vi "OutputSwerveDrive2.vi"() -> ()   [LabVIEW 2019]
doc: "This VI runs feedback and feedforward control loops, manages safety interlocks, and sends commands to the swerve drive motors."
uses:
  <vilib>/Rock Robotics/WPI/ThirdParty/Phoenix-LabVIEW/Motor Controller/Controls/CTRE_Phoenix_MotorControl_SupplyCurrentLimitConfiguration.ctl
  <vilib>/Rock Robotics/WPI/ThirdParty/Phoenix-LabVIEW/Motor Controller/Controls/CTRE_Phoenix_MotorControl_ControlMode.ctl
  <vilib>/Rock Robotics/WPI/Solenoid/WPI_SolenoidValue.ctl
  4c0f1fb3-de9e-41af-b613-55c778746a69.vi
  9255c0bb-7061-46f3-9b12-3c6a122af16e.vi
  1feddb54-1091-429e-8d95-9769f01e3028.vi
  eec0778c-44f4-445b-8f09-fbe21d33a92f.vi
  5bc46b9e-4d4b-4873-ab3e-533fd441fb60.vi
  9914bed3-0d1c-4b06-b050-22aab9a27a8c.vi
  outputs.vi
  sensors.vi
  refnums.vi
  GRNF_CTREMotor.vi
  robotprofile.vi
  <vilib>/Rock Robotics/WPI/ThirdParty/Phoenix-LabVIEW/Motor Controller/Get/CTRE_Phoenix_MotorController_GetVoltage.vi
  <vilib>/Rock Robotics/WPI/ThirdParty/Phoenix-LabVIEW/Motor Controller/Get/CTRE_Phoenix_MotorController_GetSelectedSensorData.vi
  GRNF_GenericSolenoid.vi
  dsdata.vi
  TAI_Solenoid.vi
  <vilib>/Rock Robotics/WPI/Solenoid/WPI_SolenoidSetEnum.vi
  TAI_Motor.vi
panel:
  in  "Time Below Speed (ms)":u32=500
  in  "Time Above Speed (ms)":u32=500
  in  "Switch to Low Gear (rpm)":dbl=2000.0
  in  "Switch to High Gear (rpm)":dbl=3000.0
  in  "Plotting":T1(ring)
  in  "Falcon PID":T2={"P Gain"=0.1, "I Gain"=0.0, "D Gain"=0.0, "F Gain"=0.045, "I Zone"=200.0, "Min Output"=-1.0, "Max Output"=1.0} {"Max Output" min=-1.0 max=1.0 step=0.01; "Min Output" min=-1.0 max=1.0 step=0.01; "I Zone" step=0.01; "F Gain" step=0.01; "D Gain" step=0.01; "I Gain" step=0.01; "P Gain" min=0.0 step=0.01}
  out "Controller Summary":T3(graph)
  in  "Max Speed (rpm)":dbl=6400.0
  in  "Min Speed (rpm)":dbl=10.0
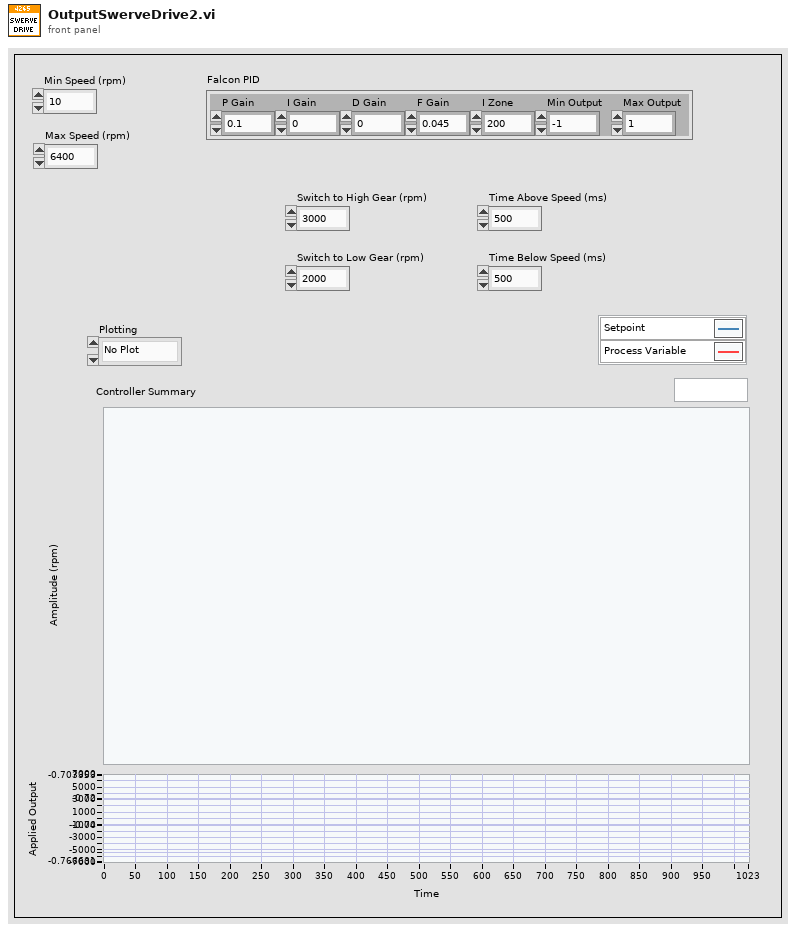
[diagram p1: front panel]
types:
  T1 = enum16{"No Plot", "Module 0", "Module 1", "Module 2", "Module 3"}
  T2 = cluster{"P Gain":dbl, "I Gain":dbl, "D Gain":dbl, "F Gain":dbl, "I Zone":dbl, "Min Output":dbl, "Max Output":dbl}
  T3 = cluster{"Sensor Velocity":dbl, "Setpoint":dbl, "Applied Output":dbl}
  T4 = typedef "CTRE_Phoenix_MotorControl_ControlMode.ctl" = u16
  T5 = typedef "CTRE_Phoenix_MotorControl_SupplyCurrentLimitConfiguration.ctl" = cluster{"Enable?":bool, "Current Limit":dbl, "Threshold Current":dbl, "Threshold Time":dbl}
  T6 = typedef "WPI_MotorControlDeviceRef.ctl" = cluster{"DeviceStatus":errorcluster, "Type":T7, "PWM":cluster{"PWM Channel":T8, "DeadBand":T9}, "CAN":cluster{"Device Number":u8, "SetOutput VI Ref":variant, "GetOutput VI Ref":variant, "Enable VI Ref":variant, "Disable VI Ref":variant, "Data":variant}, "Invert":bool, "DIO PWM":cluster{"PWM \"Enable\" Channel":T8, "DIOChannel":T10, "PWM Rate":dbl}}
  T7 = typedef "WPI_MotorControlType.ctl" = enum16{"PWM", "CAN", "DIO PWM"}
  T8 = typedef "FPGA_DIOPWMChannel.ctl" = enum8{"PWM 0", "PWM 1", "PWM 2", "PWM 3", "PWM 4", "PWM 5", "PWM 6", "PWM 7", "PWM 8", "PWM 9", "PWM MXP 0", "PWM MXP 1", "PWM MXP 2", "PWM MXP 3", "PWM MXP 4", "PWM MXP 5", "PWM MXP 6", "PWM MXP 7", "PWM MXP 8", "PWM MXP 9", "Invalid"}
  T9 = typedef "WPI_PWMDeadband.ctl" = cluster{"Name":string, "maxPositivePwm":i32, "minPositivePwm":i32, "centerPwm":i32, "maxNegativePwm":i32, "minNegativePwm":i32, "angularRange":u16}
  T10 = typedef "FPGA_DIOChannel.ctl" = enum8{"DIO 0", "DIO 1", "DIO 2", "DIO 3", "DIO 4", "DIO 5", "DIO 6", "DIO 7", "DIO 8", "DIO 9", "DIO MXP 0", "DIO MXP 1", "DIO MXP 2", "DIO MXP 3", "DIO MXP 4", "DIO MXP 5", "DIO MXP 6", "DIO MXP 7", "DIO MXP 8", "DIO MXP 9", "DIO MXP 10", "DIO MXP 11", "DIO MXP 12", "DIO MXP 13", "DIO MXP 14", "DIO MXP 15", "SPI Port CS1", "SPI Port CS2", "SPI Port CS3", "SPI Port MISO", "SPI Port MOSI", "Invalid"}
  T11 = cluster{"P Gain":bool, "I Gain":bool, "D Gain":bool, "F Gain":bool, "I Zone":bool, "Min Output":bool, "Max Output":bool}
  T12 = typedef "WPI_SolenoidValue.ctl" = enum16{"Off", "On", "Forward", "Reverse"}
  T13 = typedef "WPI_SolenoidDevRef.ctl" = cluster{"DevStatus":errorcluster, "Pneumatics Control Module":u8, "Forward Solenoid Channel":T14, "Reverse Solenoid Channel":T14}
  T14 = typedef "WPI_SolenoidChannel.ctl" = enum8{"Solenoid 0", "Solenoid 1", "Solenoid 2", "Solenoid 3", "Solenoid 4", "Solenoid 5", "Solenoid 6", "Solenoid 7", "Invalid"}
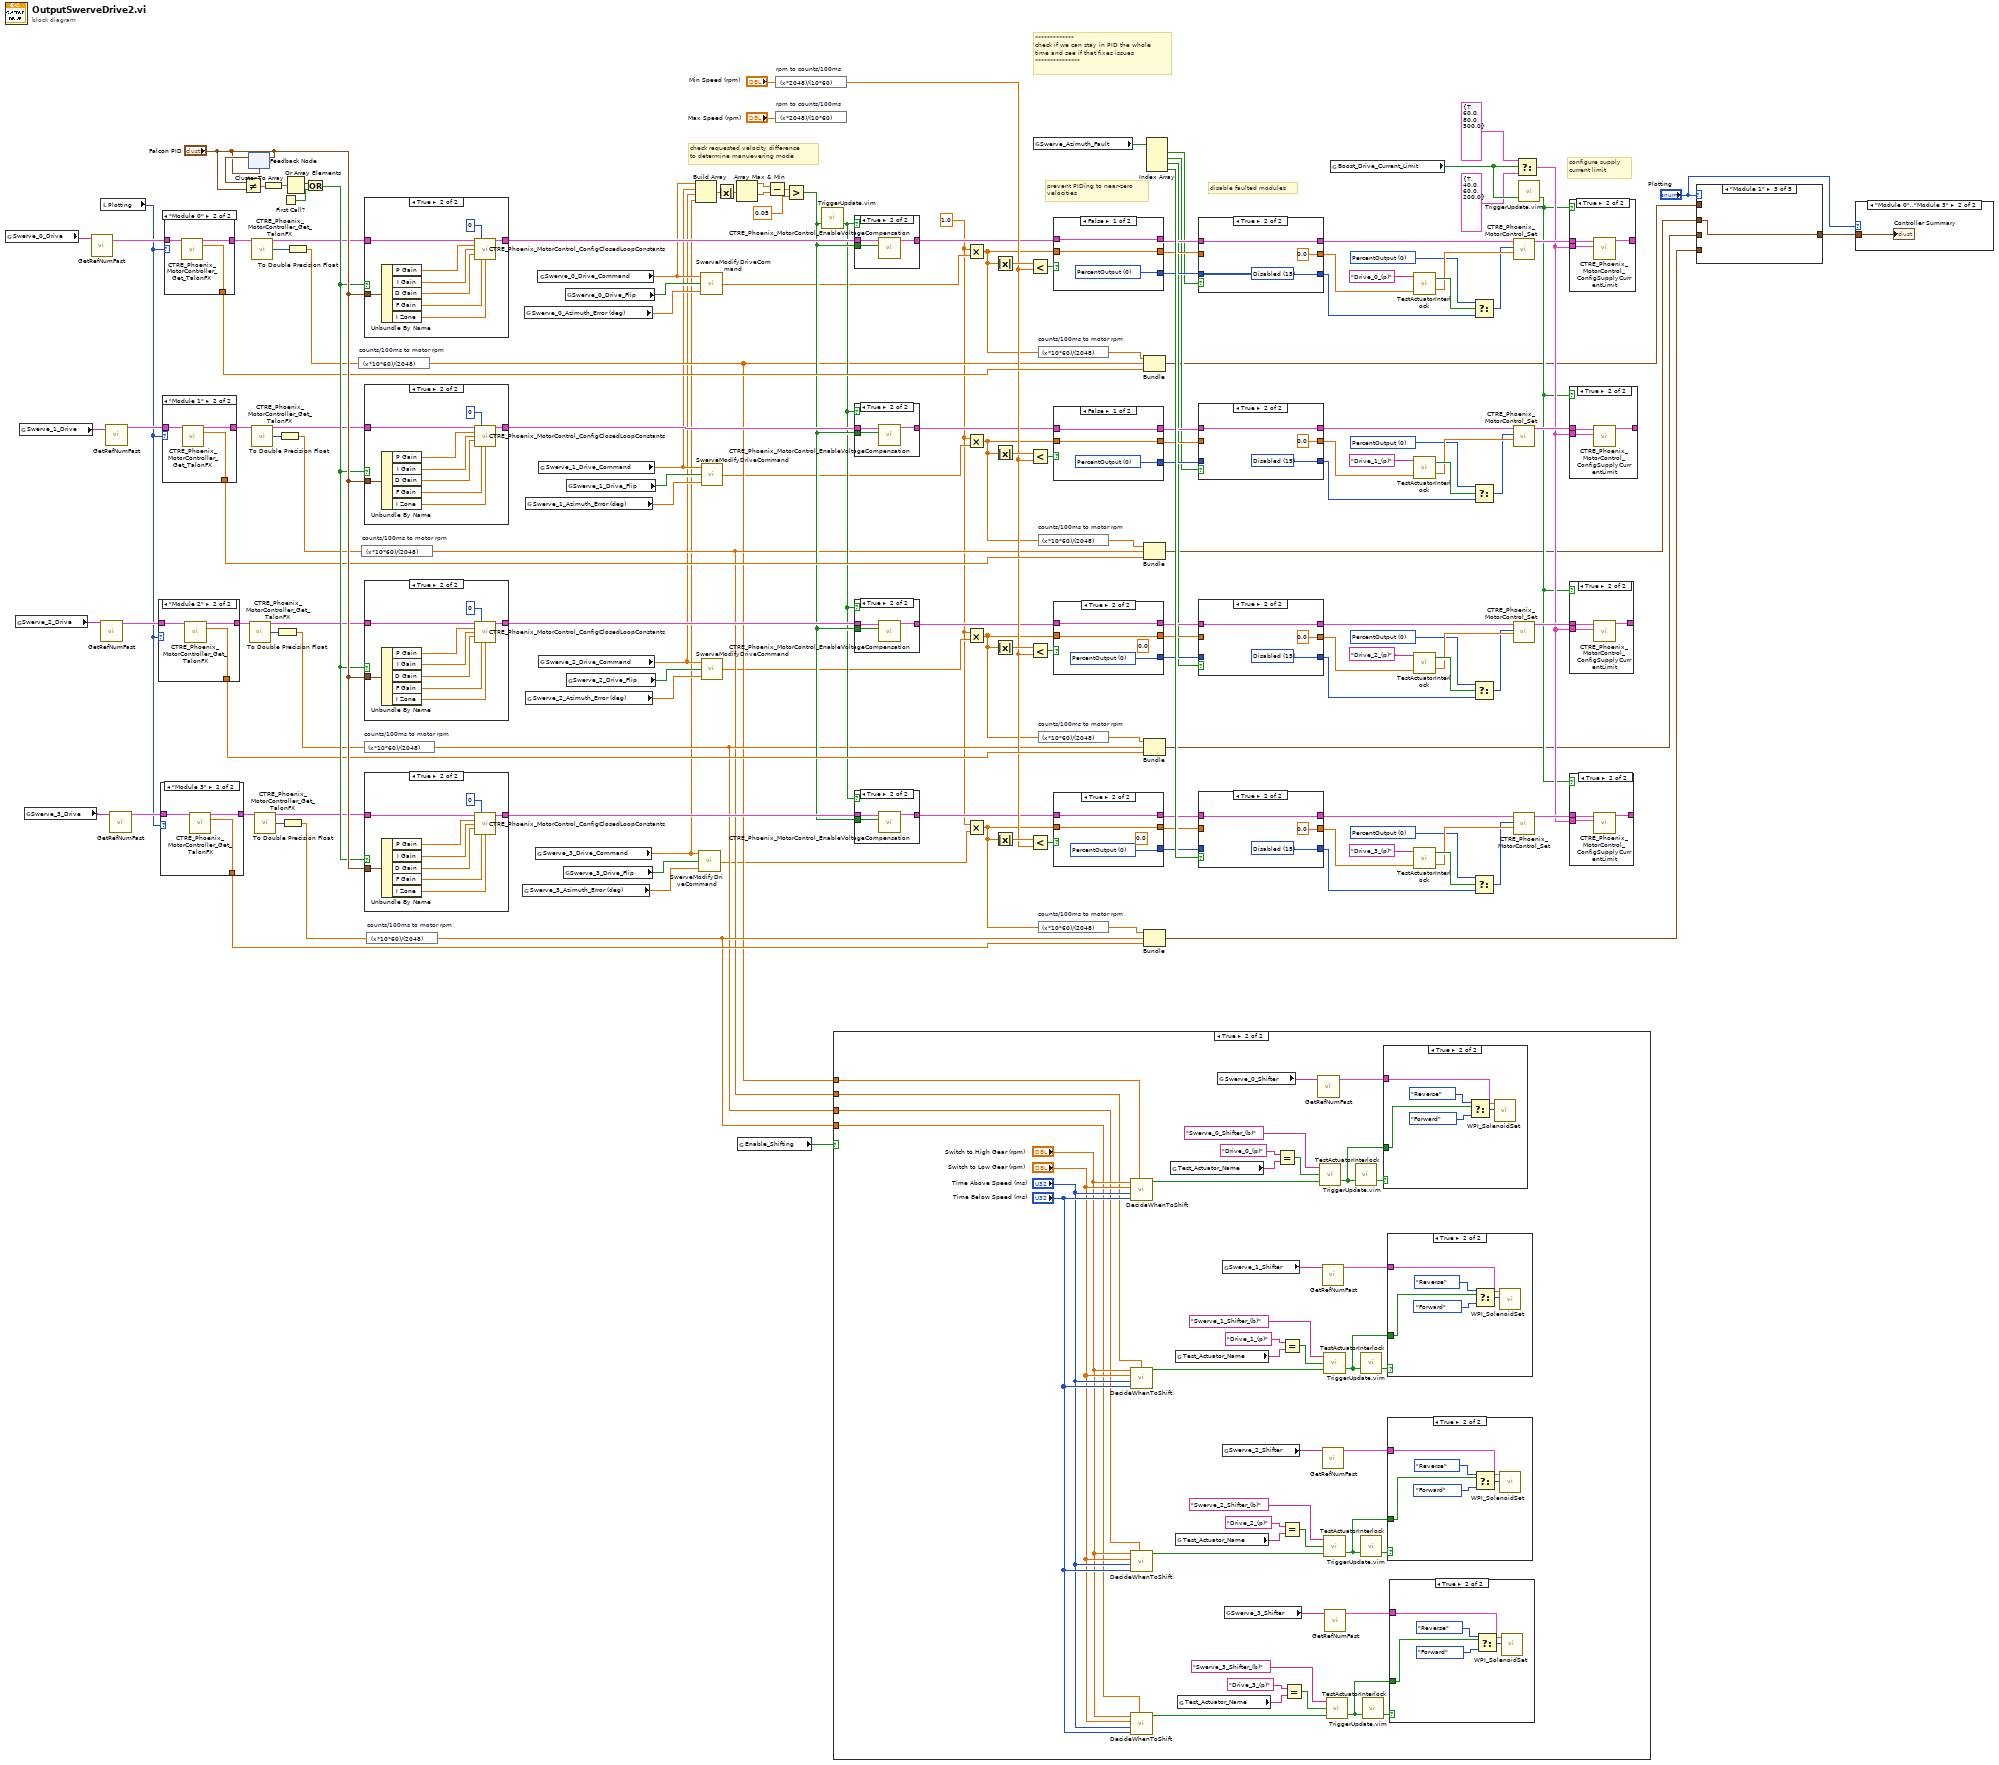
[diagram p0: block diagram]
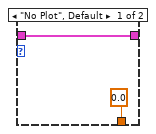
[diagram p2: hidden frame]
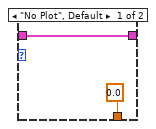
[diagram p3: hidden frame]
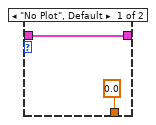
[diagram p4: hidden frame]
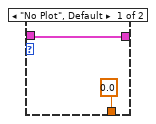
[diagram p5: hidden frame]
diagram:
  w1 = 1.0 ("x")
  w94 = T4 0 items=["PercentOutput"=0, "Position"=1, "Velocity"=2, "Current"=3, "Follower"=5, "MotionProfile"=6, "MotionMagic"=7, "MotionProfileArc"=10, "Disabled"=15] ("Control Mode")
  w108 = T4 0 items=["PercentOutput"=0, "Position"=1, "Velocity"=2, "Current"=3, "Follower"=5, "MotionProfile"=6, "MotionMagic"=7, "MotionProfileArc"=10, "Disabled"=15] ("Control Mode")
  w122 = T4 0 items=["PercentOutput"=0, "Position"=1, "Velocity"=2, "Current"=3, "Follower"=5, "MotionProfile"=6, "MotionMagic"=7, "MotionProfileArc"=10, "Disabled"=15] ("Control Mode")
  w136 = T4 0 items=["PercentOutput"=0, "Position"=1, "Velocity"=2, "Current"=3, "Follower"=5, "MotionProfile"=6, "MotionMagic"=7, "MotionProfileArc"=10, "Disabled"=15] ("Control Mode")
  # "*************\ncheck if we can stay in PID the whole \ntime and see if that fixes issues\n***************"
  # "check requested velocity difference\nto determine manuevering mode"
  # "configure supply\ncurrent limit"
  # "disable faulted modules"
  # "prevent PIDing to near-zero\nvelocities"
  n1 = global read "refnums.vi" "Swerve_0_Drive"() -> (w105:string)
  n2 = global read "refnums.vi" "Swerve_2_Drive"() -> (w133:string)
  n3 = global read "refnums.vi" "Swerve_1_Drive"() -> (w119:string)
  n4 = global read "refnums.vi" "Swerve_3_Drive"() -> (w143:string)
  n5 = call-poly "GetRefNumFast.vi"("RefNum Name"=w105) -> ("Device Reference"=w68:T6)  [unwired: 5 in, 1 out]
  n6 = local read "Plotting"() -> (w18:T1)
  n7 = call-poly "GetRefNumFast.vi"("RefNum Name"=w133) -> ("Device Reference"=w74:T6)  [unwired: 5 in, 1 out]
  n8 = call-poly "GetRefNumFast.vi"("RefNum Name"=w119) -> ("Device Reference"=w71:T6)  [unwired: 5 in, 1 out]
  n9 = call-poly "GetRefNumFast.vi"("RefNum Name"=w143) -> ("Device Reference"=w76:T6)  [unwired: 5 in, 1 out]
  n10 = case shown="\"Module 2\"" w18 {
    tunnel: [0.0 ("Percent Output") w162] -> w75
    tunnel: w74 -> [w159 w161]
    tunnel: [w159 w160] -> w21
    frame "No Plot", Default {
    }
    frame "Module 2" {
      n11 = call-poly <vilib>:"CTRE_Phoenix_MotorController_Get_TalonFX.vi"("PhoenixMotorControlDevRef"=w161) -> ("PhoenixMotorControlDevRef"=w160:T6, "Percent Output"=w162:dbl)  [unwired: 10 in, 3 out]
    }
  }
  n12 = case shown="\"Module 3\"" w18 {
    tunnel: [0.0 ("Percent Output") w167] -> w78
    tunnel: w76 -> [w164 w166]
    tunnel: [w164 w165] -> w19
    frame "No Plot", Default {
    }
    frame "Module 3" {
      n13 = call-poly <vilib>:"CTRE_Phoenix_MotorController_Get_TalonFX.vi"("PhoenixMotorControlDevRef"=w166) -> ("PhoenixMotorControlDevRef"=w165:T6, "Percent Output"=w167:dbl)  [unwired: 10 in, 3 out]
    }
  }
  n14 = case shown="\"Module 1\"" w18 {
    tunnel: [0.0 ("Percent Output") w172] -> w72
    tunnel: w71 -> [w169 w171]
    tunnel: [w169 w170] -> w23
    frame "No Plot", Default {
    }
    frame "Module 1" {
      n15 = call-poly <vilib>:"CTRE_Phoenix_MotorController_Get_TalonFX.vi"("PhoenixMotorControlDevRef"=w171) -> ("PhoenixMotorControlDevRef"=w170:T6, "Percent Output"=w172:dbl)  [unwired: 10 in, 3 out]
    }
  }
  n16 = case shown="\"Module 0\"" w18 {
    tunnel: [0.0 ("Percent Output") w177] -> w69
    tunnel: w68 -> [w174 w176]
    tunnel: [w174 w175] -> w25
    frame "No Plot", Default {
    }
    frame "Module 0" {
      n17 = call-poly <vilib>:"CTRE_Phoenix_MotorController_Get_TalonFX.vi"("PhoenixMotorControlDevRef"=w176) -> ("PhoenixMotorControlDevRef"=w175:T6, "Percent Output"=w177:dbl)  [unwired: 10 in, 3 out]
    }
  }
  n18 = feedback #1("Falcon PID") -> (w142:T2)
  n19 = Not Equal?(x=w142, y="Falcon PID") -> (x != y?=w147:T11)
  n20 = feedback-in #1("Falcon PID") -> ()
  n21 = call-poly <vilib>:"CTRE_Phoenix_MotorController_Get_TalonFX.vi"("PhoenixMotorControlDevRef"=w21) -> ("PhoenixMotorControlDevRef"=w32:T6, "Velocity (Raw Sensor Units per 100 ms)"=w22:i32)  [unwired: 11 in, 2 out]
  n22 = call-poly <vilib>:"CTRE_Phoenix_MotorController_Get_TalonFX.vi"("PhoenixMotorControlDevRef"=w25) -> ("PhoenixMotorControlDevRef"=w37:T6, "Velocity (Raw Sensor Units per 100 ms)"=w26:i32)  [unwired: 11 in, 2 out]
  n23 = call-poly <vilib>:"CTRE_Phoenix_MotorController_Get_TalonFX.vi"("PhoenixMotorControlDevRef"=w23) -> ("PhoenixMotorControlDevRef"=w34:T6, "Velocity (Raw Sensor Units per 100 ms)"=w24:i32)  [unwired: 11 in, 2 out]
  n24 = call-poly <vilib>:"CTRE_Phoenix_MotorController_Get_TalonFX.vi"("PhoenixMotorControlDevRef"=w19) -> ("PhoenixMotorControlDevRef"=w30:T6, "Velocity (Raw Sensor Units per 100 ms)"=w20:i32)  [unwired: 11 in, 2 out]
  n25 = Cluster To Array(cluster=w147) -> (array=w148:bool[])
  n26 = To Double Precision Float(number=w22) -> (double precision float=w33:dbl)
  n27 = To Double Precision Float(number=w24) -> (double precision float=w35:dbl)
  n28 = First Call?() -> (First Call?: T/F=w145:bool)
  n29 = To Double Precision Float(number=w20) -> (double precision float=w31:dbl)
  n30 = Or Array Elements(Boolean array=w148) -> (logical OR=w146:bool)
  n31 = To Double Precision Float(number=w26) -> (double precision float=w36:dbl)
  n32 = Or(x=w146, y=w145) -> (x .or. y?=w90:bool)
  n33 = expression code="(x*10*60)/(2048)" "counts/100ms to motor rpm"(w36) -> (w27:dbl)
  n34 = expression code="(x*10*60)/(2048)" "counts/100ms to motor rpm"(w35) -> (w28:dbl)
  n35 = expression code="(x*10*60)/(2048)" "counts/100ms to motor rpm"(w33) -> (w29:dbl)
  n36 = case shown="True" w90 {
    tunnel: "Falcon PID" -> [_ w186]
    tunnel: [w178 w187] -> w48
    tunnel: w37 -> [w178 w179]
    frame False {
    }
    frame True {
      n37 = Unbundle By Name(w186) -> ("P Gain"=w185:dbl, "I Gain"=w184:dbl, "D Gain"=w183:dbl, "F Gain"=w182:dbl, "I Zone"=w181:dbl)
      n38 = call <vilib>:"CTRE_Phoenix_MotorControl_ConfigClosedLoopConstants.vi"("PhoenixMotorControlDevRef"=w179, "slotIdx"=0, "P"=w185, "I"=w184, "D"=w183, "F"=w182, "I Zone"=w181) -> ("PhoenixMotorControlDevRef"=w187:T6)  [unwired: 7 in, 1 out]
    }
  }
  n39 = case shown="True" w90 {
    tunnel: w34 -> [w188 w196]
    tunnel: "Falcon PID" -> [_ w195]
    tunnel: [w188 w197] -> w46
    frame False {
    }
    frame True {
      n40 = Unbundle By Name(w195) -> ("P Gain"=w189:dbl, "I Gain"=w194:dbl, "D Gain"=w193:dbl, "F Gain"=w192:dbl, "I Zone"=w191:dbl)
      n41 = call <vilib>:"CTRE_Phoenix_MotorControl_ConfigClosedLoopConstants.vi"("PhoenixMotorControlDevRef"=w196, "slotIdx"=0, "P"=w189, "I"=w194, "D"=w193, "F"=w192, "I Zone"=w191) -> ("PhoenixMotorControlDevRef"=w197:T6)  [unwired: 7 in, 1 out]
    }
  }
  n42 = case shown="True" w90 {
    tunnel: w32 -> [w198 w206]
    tunnel: "Falcon PID" -> [_ w205]
    tunnel: [w198 w207] -> w44
    frame False {
    }
    frame True {
      n43 = Unbundle By Name(w205) -> ("P Gain"=w204:dbl, "I Gain"=w203:dbl, "D Gain"=w202:dbl, "F Gain"=w201:dbl, "I Zone"=w200:dbl)
      n44 = call <vilib>:"CTRE_Phoenix_MotorControl_ConfigClosedLoopConstants.vi"("PhoenixMotorControlDevRef"=w206, "slotIdx"=0, "P"=w204, "I"=w203, "D"=w202, "F"=w201, "I Zone"=w200) -> ("PhoenixMotorControlDevRef"=w207:T6)  [unwired: 7 in, 1 out]
    }
  }
  n45 = case shown="True" w90 {
    tunnel: w30 -> [w208 w216]
    tunnel: "Falcon PID" -> [_ w215]
    tunnel: [w208 w217] -> w42
    frame False {
    }
    frame True {
      n46 = Unbundle By Name(w215) -> ("P Gain"=w214:dbl, "I Gain"=w213:dbl, "D Gain"=w212:dbl, "F Gain"=w211:dbl, "I Zone"=w210:dbl)
      n47 = call <vilib>:"CTRE_Phoenix_MotorControl_ConfigClosedLoopConstants.vi"("PhoenixMotorControlDevRef"=w216, "slotIdx"=0, "P"=w214, "I"=w213, "D"=w212, "F"=w211, "I Zone"=w210) -> ("PhoenixMotorControlDevRef"=w217:T6)  [unwired: 7 in, 1 out]
    }
  }
  n48 = expression code="(x*10*60)/(2048)" "counts/100ms to motor rpm"(w31) -> (w63:dbl)
  n49 = global read "outputs.vi" "Swerve_3_Azimuth_Error (deg)"() -> (w4:dbl)
  n50 = global read "outputs.vi" "Swerve_0_Azimuth_Error (deg)"() -> (w15:dbl)
  n51 = global read "outputs.vi" "Swerve_1_Azimuth_Error (deg)"() -> (w12:dbl)
  n52 = global read "outputs.vi" "Swerve_2_Azimuth_Error (deg)"() -> (w8:dbl)
  n53 = global read "outputs.vi" "Swerve_3_Drive_Command"() -> (w3:dbl)
  n54 = global read "outputs.vi" "Swerve_0_Drive_Command"() -> (w16:dbl)
  n55 = global read "outputs.vi" "Swerve_1_Drive_Command"() -> (w11:dbl)
  n56 = global read "outputs.vi" "Swerve_2_Drive_Command"() -> (w7:dbl)
  n57 = global read "outputs.vi" "Swerve_3_Drive_Flip"() -> (w5:bool)
  n58 = global read "outputs.vi" "Swerve_0_Drive_Flip"() -> (w17:bool)
  n59 = global read "outputs.vi" "Swerve_1_Drive_Flip"() -> (w13:bool)
  n60 = global read "outputs.vi" "Swerve_2_Drive_Flip"() -> (w9:bool)
  n61 = Build Array(w16, w11, w7, w3) -> (w53:dbl[])
  n62 = call "SwerveModifyDriveCommand.vi"("Azimuth Error (deg)"=w4, "Flip Drive Command"=w5, "Raw Drive Command (ul)"=w3) -> ("Modified Drive Command (ul)"=w2:dbl)
  n63 = call "SwerveModifyDriveCommand.vi"("Azimuth Error (deg)"=w15, "Flip Drive Command"=w17, "Raw Drive Command (ul)"=w16) -> ("Modified Drive Command (ul)"=w14:dbl)
  n64 = call "SwerveModifyDriveCommand.vi"("Azimuth Error (deg)"=w12, "Flip Drive Command"=w13, "Raw Drive Command (ul)"=w11) -> ("Modified Drive Command (ul)"=w10:dbl)
  n65 = call "SwerveModifyDriveCommand.vi"("Azimuth Error (deg)"=w8, "Flip Drive Command"=w9, "Raw Drive Command (ul)"=w7) -> ("Modified Drive Command (ul)"=w6:dbl)
  n66 = Absolute Value(x=w53) -> (abs(x)=w38:dbl[])
  n67 = Array Max & Min(array=w38) -> (max value=w52:dbl, min value=w51:dbl)  [unwired: 2 out]
  n68 = global read "robotprofile.vi" "Enable_Shifting"() -> (w62:bool)
  n69 = Subtract(x=w52, y=w51) -> (x-y=w50:dbl)
  n70 = expression code="(x*2048)/(10*60)" "rpm to counts/100ms"("Min Speed (rpm)") -> (w65:dbl)
  n71 = expression code="(x*2048)/(10*60)" "rpm to counts/100ms"("Max Speed (rpm)") -> ()  [unwired: 1 out]
  n72 = Greater?(x=w50, y=0.05) -> (0:w40:bool)
  n73 = call "TriggerUpdate.vim"("Trigger"=w40) -> ("Update"=w39:bool)  [unwired: 2 in]
  n74 = case shown="True" w62 {
    tunnel: w63 -> [_ w219]
    tunnel: w29 -> [_ w220]
    tunnel: w28 -> [_ w218]
    tunnel: w27 -> [_ w243]
    frame False {
    }
    frame True {
      n75 = call "DecideWhenToShift.vi"("Wheel Velocity (rpm)"=w243, "Time Below Speed (ms)"="Time Below Speed (ms)", "Time Above Speed (ms)"="Time Above Speed (ms)", "Switch to Low Gear (rpm)"="Switch to Low Gear (rpm)", "Switch to High Gear (rpm)"="Switch to High Gear (rpm)") -> ("New Requested Shifter State"=w254:bool)  [unwired: 4 in]
      n76 = call "DecideWhenToShift.vi"("Wheel Velocity (rpm)"=w218, "Time Below Speed (ms)"="Time Below Speed (ms)", "Time Above Speed (ms)"="Time Above Speed (ms)", "Switch to Low Gear (rpm)"="Switch to Low Gear (rpm)", "Switch to High Gear (rpm)"="Switch to High Gear (rpm)") -> ("New Requested Shifter State"=w245:bool)  [unwired: 4 in]
      n77 = call "DecideWhenToShift.vi"("Wheel Velocity (rpm)"=w220, "Time Below Speed (ms)"="Time Below Speed (ms)", "Time Above Speed (ms)"="Time Above Speed (ms)", "Switch to Low Gear (rpm)"="Switch to Low Gear (rpm)", "Switch to High Gear (rpm)"="Switch to High Gear (rpm)") -> ("New Requested Shifter State"=w235:bool)  [unwired: 4 in]
      n78 = call "DecideWhenToShift.vi"("Wheel Velocity (rpm)"=w219, "Time Below Speed (ms)"="Time Below Speed (ms)", "Time Above Speed (ms)"="Time Above Speed (ms)", "Switch to Low Gear (rpm)"="Switch to Low Gear (rpm)", "Switch to High Gear (rpm)"="Switch to High Gear (rpm)") -> ("New Requested Shifter State"=w226:bool)  [unwired: 4 in]
      n79 = global read "dsdata.vi" "Test_Actuator_Name"() -> (w255:string)
      n80 = global read "dsdata.vi" "Test_Actuator_Name"() -> (w246:string)
      n81 = global read "dsdata.vi" "Test_Actuator_Name"() -> (w236:string)
      n82 = global read "dsdata.vi" "Test_Actuator_Name"() -> (w227:string)
      n83 = global read "refnums.vi" "Swerve_0_Shifter"() -> (w257:string)
      n84 = global read "refnums.vi" "Swerve_1_Shifter"() -> (w248:string)
      n85 = global read "refnums.vi" "Swerve_2_Shifter"() -> (w238:string)
      n86 = global read "refnums.vi" "Swerve_3_Shifter"() -> (w229:string)
      n87 = Equal?(x="Drive_0_(p)" ("Actuator_Name"), y=w255) -> (x = y?=w253:bool)
      n88 = Equal?(x="Drive_1_(p)" ("Actuator_Name"), y=w246) -> (x = y?=w244:bool)
      n89 = Equal?(x="Drive_2_(p)" ("Actuator_Name"), y=w236) -> (x = y?=w234:bool)
      n90 = Equal?(x="Drive_3_(p)" ("Actuator_Name"), y=w227) -> (x = y?=w225:bool)
      n91 = call-poly "GetRefNumFast.vi"("RefNum Name"=w257) -> ("Device Reference"=w259:T13)  [unwired: 5 in, 1 out]
      n92 = call-poly "TestActuatorInterlock.vi"("Normal Output"=w254, "Override Actuator Bypass"=w253, "Actuator Name"="Swerve_0_Shifter_(b)" ("Actuator_Name")) -> ("Interlock Output"=w260:bool)  [unwired: 1 out]
      n93 = call-poly "GetRefNumFast.vi"("RefNum Name"=w248) -> ("Device Reference"=w250:T13)  [unwired: 5 in, 1 out]
      n94 = call-poly "GetRefNumFast.vi"("RefNum Name"=w238) -> ("Device Reference"=w240:T13)  [unwired: 5 in, 1 out]
      n95 = call-poly "TestActuatorInterlock.vi"("Normal Output"=w245, "Override Actuator Bypass"=w244, "Actuator Name"="Swerve_1_Shifter_(b)" ("Actuator_Name")) -> ("Interlock Output"=w251:bool)  [unwired: 1 out]
      n96 = call-poly "TestActuatorInterlock.vi"("Normal Output"=w235, "Override Actuator Bypass"=w234, "Actuator Name"="Swerve_2_Shifter_(b)" ("Actuator_Name")) -> ("Interlock Output"=w241:bool)  [unwired: 1 out]
      n97 = call-poly "GetRefNumFast.vi"("RefNum Name"=w229) -> ("Device Reference"=w231:T13)  [unwired: 5 in, 1 out]
      n98 = call-poly "TestActuatorInterlock.vi"("Normal Output"=w226, "Override Actuator Bypass"=w225, "Actuator Name"="Swerve_3_Shifter_(b)" ("Actuator_Name")) -> ("Interlock Output"=w232:bool)  [unwired: 1 out]
      n99 = call "TriggerUpdate.vim"("Trigger"=w260) -> ("Update"=w261:bool)  [unwired: 2 in]
      n100 = call "TriggerUpdate.vim"("Trigger"=w251) -> ("Update"=w252:bool)  [unwired: 2 in]
      n101 = call "TriggerUpdate.vim"("Trigger"=w241) -> ("Update"=w242:bool)  [unwired: 2 in]
      n102 = call "TriggerUpdate.vim"("Trigger"=w232) -> ("Update"=w233:bool)  [unwired: 2 in]
      n103 = case shown="True" w261 {
        tunnel: w259 -> [_ w281]
        tunnel: w260 -> [_ w280]
        frame False {
        }
        frame True {
          n104 = Select(t=WPI_SolenoidValue."Reverse" ("Value"), s=w280, f=WPI_SolenoidValue."Forward" ("Value")) -> (s? t:f=w277:T12)
          n105 = call-poly <vilib>:"WPI_SolenoidSet.vi"("Value"=w277, "SolenoidDevRef"=w281) -> ()  [unwired: 8 in, 2 out]
        }
      }
      n106 = case shown="True" w252 {
        tunnel: w250 -> [_ w276]
        tunnel: w251 -> [_ w275]
        frame False {
        }
        frame True {
          n107 = Select(t=WPI_SolenoidValue."Reverse" ("Value"), s=w275, f=WPI_SolenoidValue."Forward" ("Value")) -> (s? t:f=w272:T12)
          n108 = call-poly <vilib>:"WPI_SolenoidSet.vi"("Value"=w272, "SolenoidDevRef"=w276) -> ()  [unwired: 8 in, 2 out]
        }
      }
      n109 = case shown="True" w242 {
        tunnel: w240 -> [_ w271]
        tunnel: w241 -> [_ w270]
        frame False {
        }
        frame True {
          n110 = Select(t=WPI_SolenoidValue."Reverse" ("Value"), s=w270, f=WPI_SolenoidValue."Forward" ("Value")) -> (s? t:f=w267:T12)
          n111 = call-poly <vilib>:"WPI_SolenoidSet.vi"("Value"=w267, "SolenoidDevRef"=w271) -> ()  [unwired: 8 in, 2 out]
        }
      }
      n112 = case shown="True" w233 {
        tunnel: w231 -> [_ w266]
        tunnel: w232 -> [_ w265]
        frame False {
        }
        frame True {
          n113 = Select(t=WPI_SolenoidValue."Reverse" ("Value"), s=w265, f=WPI_SolenoidValue."Forward" ("Value")) -> (s? t:f=w262:T12)
          n114 = call-poly <vilib>:"WPI_SolenoidSet.vi"("Value"=w262, "SolenoidDevRef"=w266) -> ()  [unwired: 8 in, 2 out]
        }
      }
    }
  }
  n115 = case shown="True" w39 {
    tunnel: w48 -> [w282 w285]
    tunnel: [w282 w284] -> w47
    tunnel: w40 -> [_ w283]
    frame False {
    }
    frame True {
      n116 = call <vilib>:"CTRE_Phoenix_MotorControl_EnableVoltageCompensation.vi"("Enable Voltage Compensation?"=w283, "PhoenixMotorControlDevRef"=w285) -> ("PhoenixMotorControlDevRef"=w284:T6)  [unwired: 8 in, 1 out]
    }
  }
  n117 = case shown="True" w39 {
    tunnel: w46 -> [w286 w289]
    tunnel: [w286 w288] -> w45
    tunnel: w40 -> [_ w287]
    frame False {
    }
    frame True {
      n118 = call <vilib>:"CTRE_Phoenix_MotorControl_EnableVoltageCompensation.vi"("Enable Voltage Compensation?"=w287, "PhoenixMotorControlDevRef"=w289) -> ("PhoenixMotorControlDevRef"=w288:T6)  [unwired: 8 in, 1 out]
    }
  }
  n119 = case shown="True" w39 {
    tunnel: w44 -> [w290 w293]
    tunnel: [w290 w292] -> w43
    tunnel: w40 -> [_ w291]
    frame False {
    }
    frame True {
      n120 = call <vilib>:"CTRE_Phoenix_MotorControl_EnableVoltageCompensation.vi"("Enable Voltage Compensation?"=w291, "PhoenixMotorControlDevRef"=w293) -> ("PhoenixMotorControlDevRef"=w292:T6)  [unwired: 8 in, 1 out]
    }
  }
  n121 = case shown="True" w39 {
    tunnel: w42 -> [w294 w297]
    tunnel: [w294 w296] -> w41
    tunnel: w40 -> [_ w295]
    frame False {
    }
    frame True {
      n122 = call <vilib>:"CTRE_Phoenix_MotorControl_EnableVoltageCompensation.vi"("Enable Voltage Compensation?"=w295, "PhoenixMotorControlDevRef"=w297) -> ("PhoenixMotorControlDevRef"=w296:T6)  [unwired: 8 in, 1 out]
    }
  }
  n123 = Multiply(x=w1, y=w14) -> (x*y=w61:dbl)
  n124 = Multiply(x=w1, y=w10) -> (x*y=w58:dbl)
  n125 = Multiply(x=w1, y=w6) -> (x*y=w56:dbl)
  n126 = Multiply(x=w1, y=w2) -> (x*y=w54:dbl)
  n127 = Absolute Value(x=w61) -> (abs(x)=w100:dbl)
  n128 = Absolute Value(x=w58) -> (abs(x)=w114:dbl)
  n129 = Absolute Value(x=w56) -> (abs(x)=w128:dbl)
  n130 = Absolute Value(x=w54) -> (abs(x)=w144:dbl)
  n131 = Less?(x=w100, y=w65) -> (x < y?=w104:bool)
  n132 = Less?(x=w114, y=w65) -> (x < y?=w118:bool)
  n133 = Less?(x=w128, y=w65) -> (x < y?=w132:bool)
  n134 = Less?(x=w144, y=w65) -> (x < y?=w152:bool)
  n135 = global read "sensors.vi" "Swerve_Azimuth_Fault"() -> (w157:bool[])
  n136 = expression code="(x*10*60)/(2048)" "counts/100ms to motor rpm"(w61) -> (w60:dbl)
  n137 = expression code="(x*10*60)/(2048)" "counts/100ms to motor rpm"(w58) -> (w59:dbl)
  n138 = expression code="(x*10*60)/(2048)" "counts/100ms to motor rpm"(w56) -> (w57:dbl)
  n139 = expression code="(x*10*60)/(2048)" "counts/100ms to motor rpm"(w54) -> (w55:dbl)
  n140 = case shown="False" w104 {
    tunnel: [w300 w303] -> w101
    tunnel: w47 -> [w300 w303]
    tunnel: [w299 w301] -> w102
    tunnel: w61 -> [w299 w301]
    tunnel: [w298 w302] -> w103
    frame False {
      w298 = T4 0 items=["PercentOutput"=0, "Position"=1, "Velocity"=2, "Current"=3, "Follower"=5, "MotionProfile"=6, "MotionMagic"=7, "MotionProfileArc"=10, "Disabled"=15] ("Control Mode")
    }
    frame True {
      w302 = T4 0 items=["PercentOutput"=0, "Position"=1, "Velocity"=2, "Current"=3, "Follower"=5, "MotionProfile"=6, "MotionMagic"=7, "MotionProfileArc"=10, "Disabled"=15] ("Control Mode")
      (unwired) 0.0 ("Command")
    }
  }
  n141 = case shown="False" w118 {
    tunnel: [w306 w309] -> w115
    tunnel: w45 -> [w306 w309]
    tunnel: [w305 w307] -> w116
    tunnel: w58 -> [w305 w307]
    tunnel: [w304 w308] -> w117
    frame False {
      w304 = T4 0 items=["PercentOutput"=0, "Position"=1, "Velocity"=2, "Current"=3, "Follower"=5, "MotionProfile"=6, "MotionMagic"=7, "MotionProfileArc"=10, "Disabled"=15] ("Control Mode")
    }
    frame True {
      w308 = T4 0 items=["PercentOutput"=0, "Position"=1, "Velocity"=2, "Current"=3, "Follower"=5, "MotionProfile"=6, "MotionMagic"=7, "MotionProfileArc"=10, "Disabled"=15] ("Control Mode")
      (unwired) 0.0 ("Command")
    }
  }
  n142 = case shown="True" w132 {
    tunnel: [w312 w315] -> w129
    tunnel: w43 -> [w312 w315]
    tunnel: [w311 w313] -> w130
    tunnel: w56 -> [w311 w313]
    tunnel: [w310 w314] -> w131
    frame False {
      w310 = T4 0 items=["PercentOutput"=0, "Position"=1, "Velocity"=2, "Current"=3, "Follower"=5, "MotionProfile"=6, "MotionMagic"=7, "MotionProfileArc"=10, "Disabled"=15] ("Control Mode")
    }
    frame True {
      w314 = T4 0 items=["PercentOutput"=0, "Position"=1, "Velocity"=2, "Current"=3, "Follower"=5, "MotionProfile"=6, "MotionMagic"=7, "MotionProfileArc"=10, "Disabled"=15] ("Control Mode")
      (unwired) 0.0 ("Command")
    }
  }
  n143 = case shown="True" w152 {
    tunnel: [w318 w321] -> w149
    tunnel: w41 -> [w318 w321]
    tunnel: [w317 w319] -> w150
    tunnel: w54 -> [w317 w319]
    tunnel: [w316 w320] -> w151
    frame False {
      w316 = T4 0 items=["PercentOutput"=0, "Position"=1, "Velocity"=2, "Current"=3, "Follower"=5, "MotionProfile"=6, "MotionMagic"=7, "MotionProfileArc"=10, "Disabled"=15] ("Control Mode")
    }
    frame True {
      w320 = T4 0 items=["PercentOutput"=0, "Position"=1, "Velocity"=2, "Current"=3, "Follower"=5, "MotionProfile"=6, "MotionMagic"=7, "MotionProfileArc"=10, "Disabled"=15] ("Control Mode")
      (unwired) 0.0 ("Command")
    }
  }
  n144 = Bundle(w60, w27, "Percent Output"=w69) -> (w67:cluster{dbl, dbl, "Percent Output":dbl})  [unwired: 1 in]
  n145 = Bundle(w59, w28, "Percent Output"=w72) -> (w70:cluster{dbl, dbl, "Percent Output":dbl})  [unwired: 1 in]
  n146 = Bundle(w57, w29, "Percent Output"=w75) -> (w73:cluster{dbl, dbl, "Percent Output":dbl})  [unwired: 1 in]
  n147 = Bundle(w55, w63, "Percent Output"=w78) -> (w79:cluster{dbl, dbl, "Percent Output":dbl})  [unwired: 1 in]
  n148 = Index Array(array=w157) -> (element #1=w89:bool, element #2=w88:bool, element #3=w87:bool, element #4=w156:bool)  [unwired: 4 in]
  n149 = case shown="True" w89 {
    tunnel: [w324 w327] -> w99
    tunnel: w101 -> [w324 w327]
    tunnel: [w323 0.0 ("Command")] -> w96
    tunnel: w102 -> [w323 _]
    tunnel: w103 -> [w322 _]
    tunnel: [w322 w325] -> w93
    frame False {
    }
    frame True {
      w325 = T4 15 items=["PercentOutput"=0, "Position"=1, "Velocity"=2, "Current"=3, "Follower"=5, "MotionProfile"=6, "MotionMagic"=7, "MotionProfileArc"=10, "Disabled"=15] ("Control Mode")
    }
  }
  n150 = case shown="True" w88 {
    tunnel: [w330 w333] -> w113
    tunnel: w115 -> [w330 w333]
    tunnel: [w329 0.0 ("Command")] -> w110
    tunnel: w116 -> [w329 _]
    tunnel: w117 -> [w328 _]
    tunnel: [w328 w331] -> w107
    frame False {
    }
    frame True {
      w331 = T4 15 items=["PercentOutput"=0, "Position"=1, "Velocity"=2, "Current"=3, "Follower"=5, "MotionProfile"=6, "MotionMagic"=7, "MotionProfileArc"=10, "Disabled"=15] ("Control Mode")
    }
  }
  n151 = case shown="True" w87 {
    tunnel: [w336 w339] -> w127
    tunnel: w129 -> [w336 w339]
    tunnel: [w335 0.0 ("Command")] -> w124
    tunnel: w130 -> [w335 _]
    tunnel: w131 -> [w334 _]
    tunnel: [w334 w337] -> w121
    frame False {
    }
    frame True {
      w337 = T4 15 items=["PercentOutput"=0, "Position"=1, "Velocity"=2, "Current"=3, "Follower"=5, "MotionProfile"=6, "MotionMagic"=7, "MotionProfileArc"=10, "Disabled"=15] ("Control Mode")
    }
  }
  n152 = case shown="True" w156 {
    tunnel: [w342 w345] -> w141
    tunnel: w149 -> [w342 w345]
    tunnel: [w341 0.0 ("Command")] -> w138
    tunnel: w150 -> [w341 _]
    tunnel: w151 -> [w340 _]
    tunnel: [w340 w343] -> w135
    frame False {
    }
    frame True {
      w343 = T4 15 items=["PercentOutput"=0, "Position"=1, "Velocity"=2, "Current"=3, "Follower"=5, "MotionProfile"=6, "MotionMagic"=7, "MotionProfileArc"=10, "Disabled"=15] ("Control Mode")
    }
  }
  n153 = global read "outputs.vi" "Boost_Drive_Current_Limit"() -> (w154:bool)
  n154 = call-poly "TestActuatorInterlock.vi"("Normal Output"=w96, "Actuator Name"="Drive_0_(p)" ("Actuator_Name")) -> ("Interlock Output"=w95:dbl, "Testing This Actuator"=w98:bool)  [unwired: 1 in]
  n155 = call-poly "TestActuatorInterlock.vi"("Normal Output"=w110, "Actuator Name"="Drive_1_(p)" ("Actuator_Name")) -> ("Interlock Output"=w109:dbl, "Testing This Actuator"=w112:bool)  [unwired: 1 in]
  n156 = call-poly "TestActuatorInterlock.vi"("Normal Output"=w124, "Actuator Name"="Drive_2_(p)" ("Actuator_Name")) -> ("Interlock Output"=w123:dbl, "Testing This Actuator"=w126:bool)  [unwired: 1 in]
  n157 = call-poly "TestActuatorInterlock.vi"("Normal Output"=w138, "Actuator Name"="Drive_3_(p)" ("Actuator_Name")) -> ("Interlock Output"=w137:dbl, "Testing This Actuator"=w140:bool)  [unwired: 1 in]
  n158 = Select(t=w94, s=w98, f=w93) -> (s? t:f=w92:T4)
  n159 = Select(t=w108, s=w112, f=w107) -> (s? t:f=w106:T4)
  n160 = Select(t=w122, s=w126, f=w121) -> (s? t:f=w120:T4)
  n161 = Select(t=w136, s=w140, f=w135) -> (s? t:f=w134:T4)
  n162 = call <vilib>:"CTRE_Phoenix_MotorControl_Set.vi"("Output"=w95, "Control Mode"=w92, "PhoenixMotorControlDevRef"=w99) -> ("PhoenixMotorControlDevRef"=w86:T6)  [unwired: 7 in, 1 out]
  n163 = call <vilib>:"CTRE_Phoenix_MotorControl_Set.vi"("Output"=w109, "Control Mode"=w106, "PhoenixMotorControlDevRef"=w113) -> ("PhoenixMotorControlDevRef"=w85:T6)  [unwired: 7 in, 1 out]
  n164 = call <vilib>:"CTRE_Phoenix_MotorControl_Set.vi"("Output"=w123, "Control Mode"=w120, "PhoenixMotorControlDevRef"=w127) -> ("PhoenixMotorControlDevRef"=w84:T6)  [unwired: 7 in, 1 out]
  n165 = call <vilib>:"CTRE_Phoenix_MotorControl_Set.vi"("Output"=w137, "Control Mode"=w134, "PhoenixMotorControlDevRef"=w141) -> ("PhoenixMotorControlDevRef"=w83:T6)  [unwired: 7 in, 1 out]
  n166 = Select(t=T5 {"Enable?"=TRUE, "Current Limit"=60.0, "Threshold Current"=80.0, "Threshold Time"=500.0} ("Supply Current Limit Configuration"), s=w154, f=T5 {"Enable?"=TRUE, "Current Limit"=40.0, "Threshold Current"=60.0, "Threshold Time"=200.0} ("Supply Current Limit Configuration")) -> (s? t:f=w82:T5)
  n167 = call "TriggerUpdate.vim"("Trigger"=w154) -> ("Update"=w81:bool)  [unwired: 2 in]
  n168 = case shown="True" w81 {
    tunnel: w86 -> [w346 w349]
    tunnel: [w346 w348] -> _
    tunnel: w82 -> [_ w347]
    frame False {
    }
    frame True {
      n169 = call <vilib>:"CTRE_Phoenix_MotorControl_ConfigSupplyCurrentLimit.vi"("Supply Current Limit Configuration"=w347, "PhoenixMotorControlDevRef"=w349) -> ("PhoenixMotorControlDevRef"=w348:T6)  [unwired: 8 in, 1 out]
    }
  }
  n170 = case shown="True" w81 {
    tunnel: w85 -> [w350 w353]
    tunnel: [w350 w352] -> _
    tunnel: w82 -> [_ w351]
    frame False {
    }
    frame True {
      n171 = call <vilib>:"CTRE_Phoenix_MotorControl_ConfigSupplyCurrentLimit.vi"("Supply Current Limit Configuration"=w351, "PhoenixMotorControlDevRef"=w353) -> ("PhoenixMotorControlDevRef"=w352:T6)  [unwired: 8 in, 1 out]
    }
  }
  n172 = case shown="True" w81 {
    tunnel: w84 -> [w354 w357]
    tunnel: [w354 w356] -> _
    tunnel: w82 -> [_ w355]
    frame False {
    }
    frame True {
      n173 = call <vilib>:"CTRE_Phoenix_MotorControl_ConfigSupplyCurrentLimit.vi"("Supply Current Limit Configuration"=w355, "PhoenixMotorControlDevRef"=w357) -> ("PhoenixMotorControlDevRef"=w356:T6)  [unwired: 8 in, 1 out]
    }
  }
  n174 = case shown="True" w81 {
    tunnel: w83 -> [w358 w361]
    tunnel: [w358 w360] -> _
    tunnel: w82 -> [_ w359]
    frame False {
    }
    frame True {
      n175 = call <vilib>:"CTRE_Phoenix_MotorControl_ConfigSupplyCurrentLimit.vi"("Supply Current Limit Configuration"=w359, "PhoenixMotorControlDevRef"=w361) -> ("PhoenixMotorControlDevRef"=w360:T6)  [unwired: 8 in, 1 out]
    }
  }
  n176 = case shown="\"Module 1\"" "Plotting" {
    tunnel: [_ w362 w363 w364 w365] -> w77
    tunnel: w70 -> [_ _ w363 _ _]
    tunnel: w73 -> [_ _ _ w364 _]
    tunnel: w79 -> [_ _ _ _ w365]
    tunnel: w67 -> [_ w362 _ _ _]
    frame "No Plot", Default {
    }
    frame "Module 0" {
    }
    frame "Module 1" {
    }
    frame "Module 2" {
    }
    frame "Module 3" {
    }
  }
  n177 = case shown="\"Module 0\"..\"Module 3\"" "Plotting" {
    tunnel: w77 -> [_ w366]
    frame "No Plot", Default {
    }
    frame "Module 0".."Module 3" {
      "Controller Summary" <- w366
    }
  }
